vi "Test-PlayerVsComputerNoGuesses.vi"() -> ()   [LabVIEW 2017]
panel:
  out "Result":string
  in  "stop":bool
  in  "Guess":bool
  in  "Number":i32 caption="Guess"
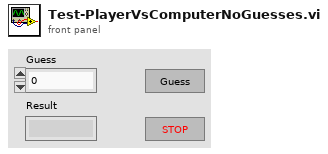
[diagram p1: front panel]
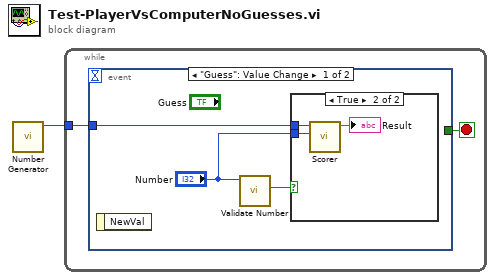
[diagram p0: block diagram]
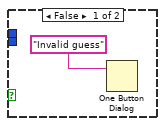
[diagram p2: hidden frame]
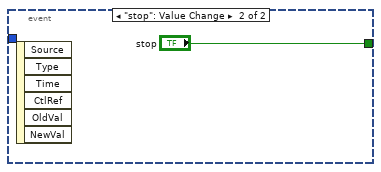
[diagram p3: hidden frame]
diagram:
  n1 = call "Number Generator.vi"() -> ("Random Number"=w1:i32)  [unwired: 11 in]
  n2 = while {
    tunnel: w1 -> [w3]
    stop <- w2 stop-if-true
    n3 = event shown="[0] \"Guess\": Value Change" {
      selector: _ -> [_ _]
      dyn-events: _ -> [_ _]
      timeout: _ -> [_ _]
      tunnel: w3 -> [w6 _]
      tunnel: [_ "stop"] -> w2
      event "Guess": Value Change {
        n4 = event-data() -> ()  [unwired: 1 in, 1 out]
        n5 = call "Validate Number.vi"("Number"="Number") -> ("Valid?"=w4:bool)  [unwired: 9 in, 1 out]
        n6 = case shown="True" w4 {
          tunnel: w6 -> [_ w10]
          tunnel: "Number" -> [_ w9]
          frame False {
            n7 = One Button Dialog(message="Invalid guess") -> ()  [unwired: 1 in, 1 out]
          }
          frame True {
            n8 = call "Scorer.vi"("Guess"=w9, "Answer"=w10) -> ("Result"=→"Result":string)  [unwired: 6 in, 3 out]
          }
        }
      }
      event "stop": Value Change {
        n9 = event-data() -> ()  [unwired: 1 in, 6 out]
      }
    }
  }
